vi "LCA Lookup Axis System By Name.vi"(8 "error in (no error)":errorcluster caption="Fehler (Eingang, kein Fehler)", 11 "Axis System Name":string) -> (0 "error out":errorcluster caption="Fehler (Ausgang)", 3 "Axis System Handle":i64)   [LabVIEW 2021, in "labbCAN_MotionControl_API.lvlib"]
doc: "LCA_Func dev_hdl __stdcall LCA_LookupAxisSystemByName(const char *pAxisName);"
uses:
  labbCAN_MotionControl_API.lvlib
  labbCAN_MotionControl_API.dll
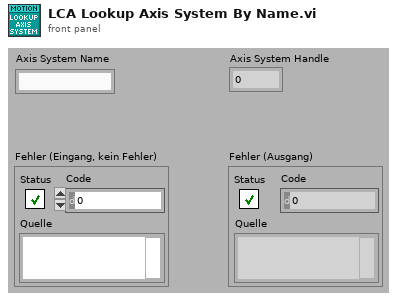
[diagram p1: front panel]
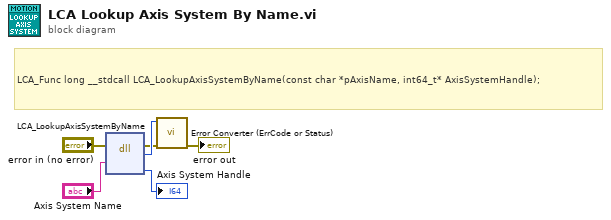
[diagram p0: block diagram]
diagram:
  # "LCA_Func long __stdcall LCA_LookupAxisSystemByName(const char *pAxisName, int64_t* AxisSystemHandle);"
  n1 = dll-call lib="C:/Users/olaja/AppData/Local/CETONI_SDK/labbCAN_MotionControl_API.*" fn="LCA_LookupAxisSystemByName"(error in="error in (no error)", "pAxisName"="Axis System Name") -> (error out=w3:errorcluster, "Rückgabetyp"=w6:i32, "AxisSystemHandle"=→"Axis System Handle":i64)  [unwired: 4 in, 1 out]
  n2 = call "Error Converter (ErrCode or Status).vi"("error in (no error)"=w3, "error code"=w6) -> ("error out"=→"error out":errorcluster)  [unwired: 9 in]
